vi "2Darray to FlattenedData1Darray.vi"(7 "2D array":dbl[][](array[numeric])) -> (3 "Flattened data 1D array":T1[](array[typedef]))   [LabVIEW 2020, in "SignalConverson.lvlib"]
uses:
  SignalConverson.lvlib
  FlattenedData.ctl
panel:
  in  "Flattened data":T1
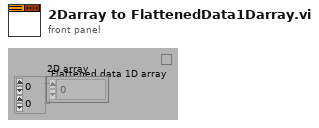
[diagram p1: front panel]
types:
  T1 = typedef "SignalConverson.lvlib/FlattenedData.ctl" = cluster{"V_A' [V]":dbl, "V_D' [V]":dbl, "V_P'  [V]":dbl, "V_S' [V]":dbl, "V_L' [V]":dbl, "V_R' [V]":dbl, "V_sum' [V]":dbl, "V_x [V]":dbl, "V_y [V]":dbl, "V_px' [V]":dbl, "V_py' [V]":dbl, "V_pz' [V]":dbl, "dt [s]":dbl, "Vpx_AO [V]":dbl, "Vpy_AO [V]":dbl, "Vpz_AO [V]":dbl, "scan backlog":dbl, "LockInPhase":dbl, "TrapX [nm]":dbl, "TrapY [nm]":dbl, "TrapZ [nm]":dbl, "V_A [V]":dbl, "V_D [V]":dbl, "V_P [V]":dbl, "V_S [V]":dbl, "V_L [V]":dbl, "V_R [V]":dbl, "V_sum [V]":dbl, "V_x [V]":dbl, "V_y [V]":dbl, "P power [mW]":dbl, "S power [mW]":dbl, "angle compensated P power [W]":dbl, "angle compensated S power [W]":dbl, "angle compensated V_L":dbl, "angle compensated V_R":dbl, "angle compensated V_sum [V]":dbl, "angle compensated V_x [V]":dbl, "angle compensated V_y [V]":dbl, "Psi [rad]":dbl, "Laser power before objective[W]":dbl, "E_in":dbl, "E_out":dbl, "Delta E":dbl, "X signal":dbl, "Y signal":dbl, "Z signal":dbl, "TrapX (AO) [nm]":dbl, "TrapY (AO) [nm]":dbl, "TrapZ (AO) [nm]":dbl, "Fz [pN]":dbl, "Zext [nm]":dbl, "Tau [pNnm]":dbl, "Turn":dbl, "Fx [pN]":dbl, "Xext [nm]":dbl, "Fy [pN]":dbl, "Yext [nm]":dbl, "time [s]":dbl, "Delta Z signal":dbl, "Delta Z bead [nm]":dbl, "Z bead [nm]":dbl, "Delta TrapZ [nm]":dbl, "Delta Xsignal":dbl, "X bead [nm]":dbl, "Delta Ysignal":dbl, "Y bead [nm]":dbl, "Stop Condition":dbl}
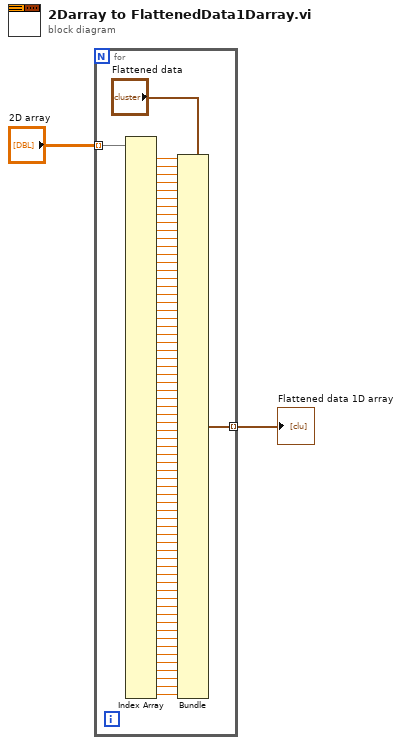
[diagram p0: block diagram]
diagram:
  n1 = for {
    tunnel: "2D array" -> [w58] mode=indexing
    tunnel: [w3] -> w1 mode=indexing
    n2 = Index Array(array=w58) -> (element #1=w73:dbl, element #2=w72:dbl, element #3=w71:dbl, element #4=w70:dbl, element #5=w69:dbl, element #6=w68:dbl, element #7=w67:dbl, element #8=w66:dbl, element #9=w65:dbl, element #10=w64:dbl, element #11=w63:dbl, element #12=w62:dbl, element #13=w61:dbl, element #14=w60:dbl, element #15=w59:dbl, element #16=w57:dbl, element #17=w56:dbl, element #18=w55:dbl, element #19=w54:dbl, element #20=w53:dbl, element #21=w52:dbl, element #22=w51:dbl, element #23=w50:dbl, element #24=w49:dbl, element #25=w48:dbl, element #26=w47:dbl, element #27=w46:dbl, element #28=w45:dbl, element #29=w44:dbl, element #30=w43:dbl, element #31=w42:dbl, element #32=w41:dbl, element #33=w40:dbl, element #34=w39:dbl, element #35=w38:dbl, element #36=w37:dbl, element #37=w36:dbl, element #38=w35:dbl, element #39=w34:dbl, element #40=w33:dbl, element #41=w32:dbl, element #42=w31:dbl, element #43=w30:dbl, element #44=w29:dbl, element #45=w28:dbl, element #46=w27:dbl, element #47=w26:dbl, element #48=w25:dbl, element #49=w24:dbl, element #50=w23:dbl, element #51=w22:dbl, element #52=w21:dbl, element #53=w20:dbl, element #54=w19:dbl, element #55=w18:dbl, element #56=w17:dbl, element #57=w16:dbl, element #58=w15:dbl, element #59=w14:dbl, element #60=w13:dbl, element #61=w12:dbl, element #62=w11:dbl, element #63=w10:dbl, element #64=w9:dbl, element #65=w7:dbl, element #66=w6:dbl, element #67=w5:dbl, element #68=w4:dbl)  [unwired: 68 in]
    n3 = Bundle(cluster="Flattened data", "V_A' [V]"=w73, "V_D' [V]"=w72, "V_P'  [V]"=w71, "V_S' [V]"=w70, "V_L' [V]"=w69, "V_R' [V]"=w68, "V_sum' [V]"=w67, "V_x [V]"=w66, "V_y [V]"=w65, "V_px' [V]"=w64, "V_py' [V]"=w63, "V_pz' [V]"=w62, "dt [s]"=w61, "Vpx_AO [V]"=w60, "Vpy_AO [V]"=w59, "Vpz_AO [V]"=w57, "scan backlog"=w56, "LockInPhase"=w55, "TrapX [nm]"=w54, "TrapY [nm]"=w53, "TrapZ [nm]"=w52, "V_A [V]"=w51, "V_D [V]"=w50, "V_P [V]"=w49, "V_S [V]"=w48, "V_L [V]"=w47, "V_R [V]"=w46, "V_sum [V]"=w45, "V_x [V]"=w44, "V_y [V]"=w43, "P power [mW]"=w42, "S power [mW]"=w41, "angle compensated P power [W]"=w40, "angle compensated S power [W]"=w39, "angle compensated V_L"=w38, "angle compensated V_R"=w37, "angle compensated V_sum [V]"=w36, "angle compensated V_x [V]"=w35, "angle compensated V_y [V]"=w34, "Psi [rad]"=w33, "Laser power before objective[W]"=w32, "E_in"=w31, "E_out"=w30, "Delta E"=w29, "X signal"=w28, "Y signal"=w27, "Z signal"=w26, "TrapX (AO) [nm]"=w25, "TrapY (AO) [nm]"=w24, "TrapZ (AO) [nm]"=w23, "Fz [pN]"=w22, "Zext [nm]"=w21, "Tau [pNnm]"=w20, "Turn"=w19, "Fx [pN]"=w18, "Xext [nm]"=w17, "Fy [pN]"=w16, "Yext [nm]"=w15, "time [s]"=w14, "Delta Z signal"=w13, "Delta Z bead [nm]"=w12, "Z bead [nm]"=w11, "Delta TrapZ [nm]"=w10, "Delta Xsignal"=w9, "X bead [nm]"=w7, "Delta Ysignal"=w6, "Y bead [nm]"=w5, "Stop Condition"=w4) -> (w3:T1)
  }
  "Flattened data 1D array" <- w1
